vi "GlobalDataNames.vi"() -> ()   [LabVIEW 2019]
panel:
  in  "stringDataNames":string="stringDataNames"
  in  "stringData":string="stringData"
  in  "numDataNames":string="numDataNames"
  in  "numData":string="numData"
  in  "boolDataNames":string="boolDataNames"
  in  "boolData":string="boolData"
  in  "stringCalDataNames":string="stringCalDataNames"
  in  "stringCalData":string="stringCalData"
  in  "numCalDataNames":string="numCalDataNames"
  in  "numCalData":string="numCalData"
  in  "boolCalDataNames":string="boolCalDataNames"
  in  "boolCalData":string="boolCalData"
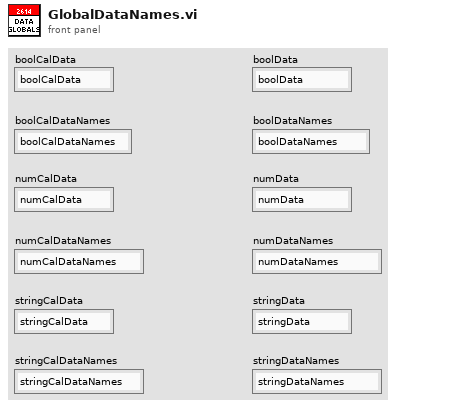
[diagram p1: front panel]
diagram:
